vi "SubscribedMessages.vi"() -> (3 "subscribed messages":string[](array[string]))   [LabVIEW 2017, in "BurstMode.lvlib"]
uses:
  <vilib>/addons/InsightCM/Devices/Shared/Cms/CmsBurstMode/BurstMode.lvlib
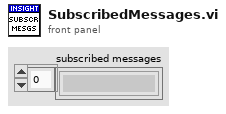
[diagram p1: front panel]
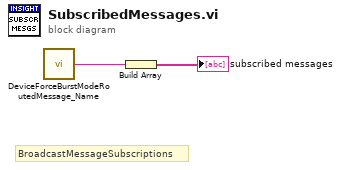
[diagram p0: block diagram]
diagram:
  # "BroadcastMessageSubscriptions"
  n1 = call <vilib>:"DeviceForceBurstModeRoutedMessage_Name.vi"() -> ("MessageName"=w1:string)  [unwired: 5 in]
  n2 = Build Array(w1) -> (→"subscribed messages":string[])
